vi "WriteToStageFIFOs.vi"(5 "Stage":T1, 7 "Enable":bool, 8 "ScaleMeas":fxp<+/-,16,1>, 9 "Scale4-7":fxp<+/-,24,1>, 10 "Scale1":fxp<+/-,18,1>, 11 "Digitiz":fxp<+/-,16,16>) -> ()   [LabVIEW 2018]
uses:
  FPGA_Controls/FilterStageEnum.ctl
  <vilib>/rvi/interface/RandomDataEmulation/niFpgaRandomDataHandleErrors.vi
  <vilib>/rvi/DataTransferAndStorage/Container/XNode/niFpgaContainer.xnode
  <vilib>/rvi/interface/RandomDataEmulation/nirviRandomDataFpgaReadWriteTemplate.vi
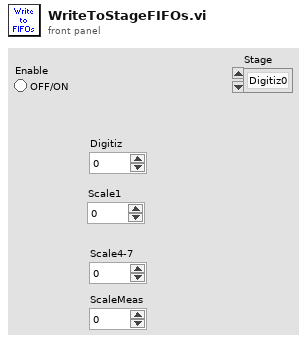
[diagram p1: front panel]
types:
  T1 = typedef "FilterStageEnum.ctl" = enum16{"Digitiz0", "Digitiz1", "ScaleMeas", "Scale1", "Scale4", "Scale5", "Scale6", "Scale7"}
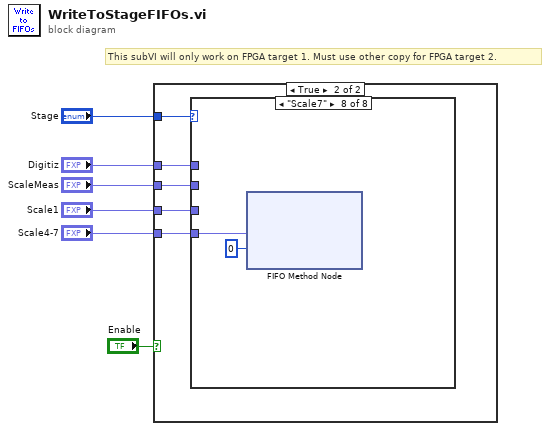
[diagram p0: block diagram]
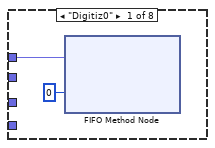
[diagram p3: hidden frame]
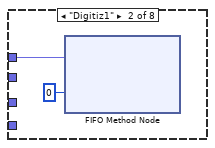
[diagram p4: hidden frame]
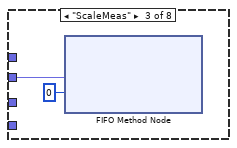
[diagram p5: hidden frame]
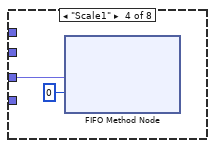
[diagram p6: hidden frame]
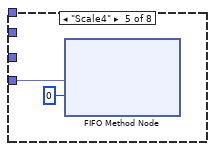
[diagram p7: hidden frame]
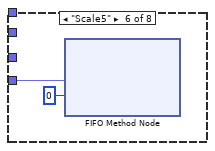
[diagram p8: hidden frame]
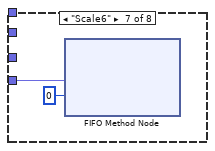
[diagram p9: hidden frame]
diagram:
  # "This subVI will only work on FPGA target 1. Must use other copy for FPGA target 2."
  n1 = case shown="True" "Enable" {
    tunnel: "Stage" -> [_ w11]
    tunnel: "Digitiz" -> [_ w10]
    tunnel: "Scale1" -> [_ w9]
    tunnel: "Scale4-7" -> [_ w8]
    tunnel: "ScaleMeas" -> [_ w7]
    frame False {
    }
    frame True {
      n2 = case shown="\"Scale7\"" w11 {
        tunnel: w10 -> [w13 w15 _ _ _ _ _ _]
        tunnel: w9 -> [_ _ _ w19 _ _ _ _]
        tunnel: w8 -> [_ _ _ _ w21 w23 w25 w27]
        tunnel: w7 -> [_ _ w16 _ _ _ _ _]
        frame "Digitiz0" {
          n3 = xnode ("FIFO Method Node")("Element"=w13, "Timeout"=0) -> ()  [unwired: 1 in, 2 out]
        }
        frame "Digitiz1" {
          n4 = xnode ("FIFO Method Node")("Element"=w15, "Timeout"=0) -> ()  [unwired: 1 in, 2 out]
        }
        frame "ScaleMeas" {
          n5 = xnode ("FIFO Method Node")("Element"=w16, "Timeout"=0) -> ()  [unwired: 1 in, 2 out]
        }
        frame "Scale1" {
          n6 = xnode ("FIFO Method Node")("Element"=w19, "Timeout"=0) -> ()  [unwired: 1 in, 2 out]
        }
        frame "Scale4" {
          n7 = xnode ("FIFO Method Node")("Element"=w21, "Timeout"=0) -> ()  [unwired: 1 in, 2 out]
        }
        frame "Scale5" {
          n8 = xnode ("FIFO Method Node")("Element"=w23, "Timeout"=0) -> ()  [unwired: 1 in, 2 out]
        }
        frame "Scale6" {
          n9 = xnode ("FIFO Method Node")("Element"=w25, "Timeout"=0) -> ()  [unwired: 1 in, 2 out]
        }
        frame "Scale7" {
          n10 = xnode ("FIFO Method Node")("Element"=w27, "Timeout"=0) -> ()  [unwired: 1 in, 2 out]
        }
      }
    }
  }
